vi "Generate_WayPoints_Hopping_CV_RunningAverage.vi"(11 "Input Cluster":T2={"Scan Rate (um/s)"=15.0, "X Start"=15.0, "X End"=15.0, "Y Start"=15.0, "Y End"=15.0, " Z Start"=15.0, "HoppingDistance"=1.0, "V"=15.0, "Z End"=15.0, "Approach Rate Hopping (um/s)"=15.0, "Retrack Rate (um/s)"=15.0, "V 2"=15.0, "Approach Rate (um/s)"=15.0, "V 3"=15.0, "CV Rate / V/s"=15.0, "V 4"=15.0, "V 1"=15.0, "HoldTime1/s"=15.0, "Hold time 2 / s"=15.0, "Hold time 3/ s"=15.0}) -> (0 "output cluster":T1)   [LabVIEW 2023]
uses:
  TypeDefs/WayPointCluster.ctl
  User_Vi/Settings.vi
panel:
  in  "WayPointCluster":T1
  out "Y  P":dbl
  out "X  P":dbl
  out "HoppingDistanceX":dbl
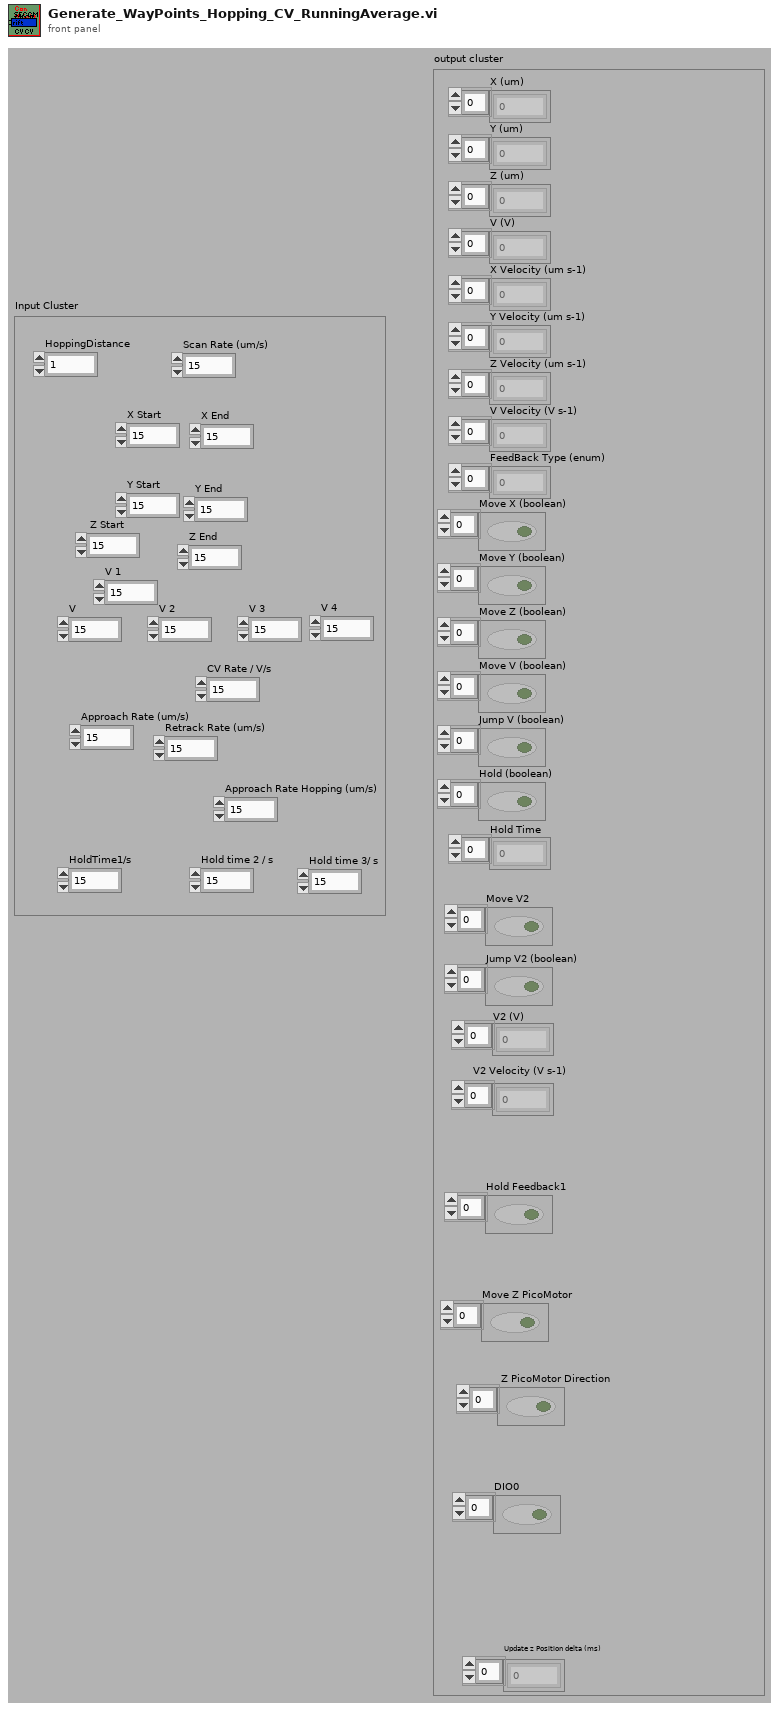
[diagram p1: front panel]
types:
  T1 = typedef "WayPointCluster.ctl" = cluster{"X (um)":dbl[], "Y (um)":dbl[], "Z (um)":dbl[], "V (V)":dbl[], "X Velocity (um s-1)":dbl[], "Y Velocity (um s-1)":dbl[], "Z Velocity (um s-1)":dbl[], "V Velocity (V s-1)":dbl[], "FeedBack Type (enum)":u16[], "Move X (boolean)":bool[], "Move Y (boolean)":bool[], "Move Z (boolean)":bool[], "Move V (boolean)":bool[], "Jump V (boolean)":bool[], "Hold (boolean)":bool[], "Hold Time":u32[], "V2 (V)":dbl[], "Move V2":bool[], "V2 Velocity (V s-1)":dbl[], "Jump V2 (boolean)":bool[], "Update z Position delta (ms)":i16[], "Hold Feedback1":bool[], "Move Z PicoMotor":bool[], " Z PicoMotor Direction":bool[], "DIO0":bool[]}
  T2 = cluster{"Scan Rate (um/s)":dbl, "X Start":dbl, "X End":dbl, "Y Start":dbl, "Y End":dbl, " Z Start":dbl, "HoppingDistance":dbl, "V":dbl, "Z End":dbl, "Approach Rate Hopping (um/s)":dbl, "Retrack Rate (um/s)":dbl, "V 2":dbl, "Approach Rate (um/s)":dbl, "V 3":dbl, "CV Rate / V/s":dbl, "V 4":dbl, "V 1":dbl, "HoldTime1/s":dbl, "Hold time 2 / s":dbl, "Hold time 3/ s":dbl}
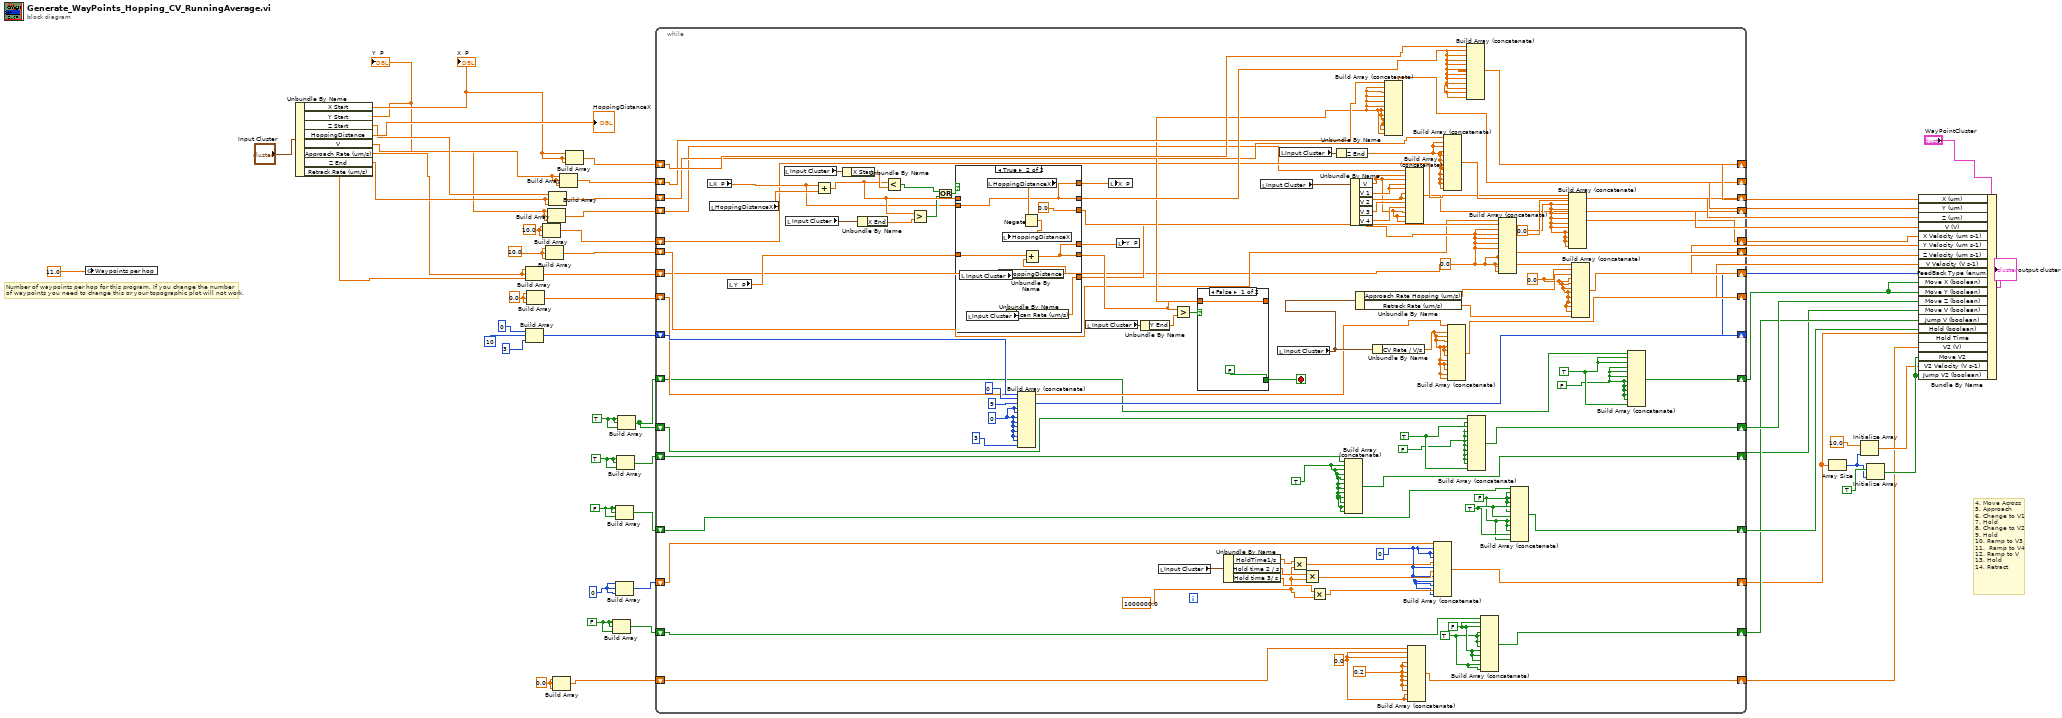
[diagram p0: block diagram]
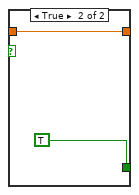
[diagram p2: hidden frame]
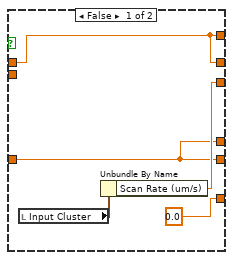
[diagram p3: hidden frame]
diagram:
  w4 = 0.0 ("element")
  w21 = FALSE
  w25 = FALSE
  w24 = u32 0 ("element")
  w23 = TRUE
  w19 = TRUE
  w15 = 10.0 ("element")
  w16 = 10.0 ("element")
  w18 = 0.0 ("element")
  # "Number of waypoints per hop for this program. If you change the number\nof waypoints you need to change this or your topographic plot will not work."
  # "4. Move Across\n5. Approach\n6. Change to V1\n7. Hold\n8. Change to V2\n9. Hold\n10. Ramp to V3\n11.  Ramp to V4\n12. Ramp to V\n13. Hold\n14. Retract"
  n1 = global write "Settings.vi" "Waypoints per hop"(11.0) -> ()
  n2 = Unbundle By Name("Input Cluster") -> ("X Start"=w39:dbl, "Y Start"=w38:dbl, "Z Start"=w40:dbl, "HoppingDistance"=→"HoppingDistanceX":dbl, "V"=w36:dbl, "Approach Rate (um/s)"=w17:dbl, "Z End"=w37:dbl, "Retrack Rate (um/s)"=w35:dbl)
  "X  P" <- w39
  "Y  P" <- w38
  n3 = Build Array(w17, w17, w35) -> (w47:dbl[])
  n4 = Build Array(u16 0 ("element"), u16 10 ("element"), u16 3 ("element")) -> (w43:u16[])
  n5 = Build Array(w18, w18, w18) -> (w45:dbl[])
  n6 = Build Array(w15, w15, w15) -> (w50:dbl[])
  n7 = Build Array(w16, w16, w16) -> (w49:dbl[])
  n8 = Build Array(w36, w36, w36) -> (w52:dbl[])
  n9 = Build Array(w40, w37, w37) -> (w54:dbl[])
  n10 = Build Array(w4, w4, w4) -> (w3:dbl[])
  n11 = Build Array(w38, w38, w38) -> (w56:dbl[])
  n12 = Build Array(w39, w39, w39) -> (w58:dbl[])
  n13 = Build Array(w25, w25, w25) -> (w29:bool[])
  n14 = Build Array(w21, w21, w21) -> (w20:bool[])
  n15 = Build Array(w24, w24, w24) -> (w32:u32[])
  n16 = Build Array(w23, w23, w23) -> (w27:bool[])
  n17 = Build Array(w19, w19, w19) -> (w11:bool[])
  n18 = while {
    shift-right: [w125] -> w57
    shift-left: w58 -> [w126]
    shift-right: [w122] -> w55
    shift-left: w56 -> [w123]
    shift-right: [w119] -> w53
    shift-left: w54 -> [w120]
    shift-right: [w109] -> w51
    shift-left: w52 -> [w110]
    shift-right: [w103] -> w33
    shift-left: w50 -> [w117]
    shift-right: [w112] -> w48
    shift-left: w49 -> [w113]
    shift-right: [w101] -> w46
    shift-left: w47 -> [w102]
    shift-right: [w96] -> w44
    shift-left: w45 -> [w97]
    shift-right: [w149] -> w42
    shift-left: w43 -> [w150]
    shift-right: [w93] -> w31
    shift-left: w11 -> [w94]
    shift-right: [w87] -> w30
    shift-left: w20 -> [w88]
    shift-right: [w83] -> w10
    shift-left: w32 -> [w84]
    shift-right: [w73] -> w28
    shift-left: w29 -> [w74]
    shift-right: [w90] -> w22
    shift-left: w27 -> [w91]
    shift-right: [w66] -> w12
    shift-left: w11 -> [w65]
    shift-right: [w63] -> w2
    shift-left: w3 -> [w64]
    stop <- w137 stop-if-true
    w62 = 0.2 ("element")
    w61 = 0.0 ("element")
    w68 = FALSE
    w69 = TRUE
    w70 = 1000000.0 ("y")
    w71 = TRUE
    w115 = 0.0 ("element")
    w89 = TRUE
    w72 = FALSE
    w75 = u32 0 ("element")
    w86 = TRUE
    w85 = FALSE
    w67 = FALSE
    w92 = TRUE
    w128 = u16 0 ("element")
    w111 = 0.0 ("element")
    w99 = 0.0 ("element")
    n19 = local read "X  P"() -> (w136:dbl)
    n20 = local read "HoppingDistanceX"() -> (w151:dbl)
    n21 = local read "Y  P"() -> (w135:dbl)
    n22 = local read "Input Cluster"() -> (w153:T2)
    n23 = local read "Input Cluster"() -> (w152:T2)
    n24 = Add(x=w136, y=w151) -> (x+y=w143:dbl)
    n25 = Unbundle By Name(w153) -> ("X Start"=w146:dbl)
    n26 = Unbundle By Name(w152) -> ("X End"=w144:dbl)
    n27 = Less?(x=w143, y=w146) -> (x < y?=w145:bool)
    n28 = Greater?(x=w143, y=w144) -> (0:w142:bool)
    n29 = Or(x=w145, y=w142) -> (x .or. y?=w141:bool)
    n30 = case shown="True" w141 {
      tunnel: w143 -> [w158 _]
      tunnel: [w158 w164] -> w124
      tunnel: w136 -> [_ w164]
      tunnel: w135 -> [w159 w165]
      tunnel: [w159 w163] -> w134
      tunnel: [w161 0.0] -> w116
      tunnel: [0.0 w166] -> w114
      tunnel: [w159 w163] -> w133
      tunnel: [w158 w164] -> w132
      frame False {
        n31 = local read "Input Cluster"() -> (w162:T2)
        n32 = Unbundle By Name(w162) -> ("Scan Rate (um/s)"=w161:dbl)
      }
      frame True {
        n33 = local read "Input Cluster"() -> (w170:T2)
        n34 = local read "Input Cluster"() -> (w168:T2)
        n35 = local read "HoppingDistanceX"() -> (w172:dbl)
        n36 = Unbundle By Name(w170) -> ("HoppingDistance"=w169:dbl)
        n37 = Unbundle By Name(w168) -> ("Scan Rate (um/s)"=w166:dbl)
        n38 = Negate(x=w172) -> (-x=w171:dbl)
        n39 = local write "HoppingDistanceX"(w171) -> ()
        n40 = Add(x=w165, y=w169) -> (x+y=w163:dbl)
      }
    }
    n41 = Build Array (concatenate)(w150, u16 0 ("element"), u16 9 ("element"), w128, w128, w128, w128, w128, w128, w128, w128, u16 3 ("element")) -> (w149:u16[])
    n42 = local read "Input Cluster"() -> (w140:T2)
    n43 = local write "X  P"(w132) -> ()
    n44 = local write "Y  P"(w133) -> ()
    n45 = Unbundle By Name(w140) -> ("Y End"=w139:dbl)
    n46 = local read "Input Cluster"() -> (w82:T2)
    n47 = Greater?(x=w134, y=w139) -> (0:w138:bool)
    n48 = case shown="False" w138 {
      tunnel: w134 -> [w155 w157]
      tunnel: [w155 w157] -> w121
      tunnel: [FALSE TRUE] -> w137
      frame False {
      }
      frame True {
      }
    }
    n49 = Unbundle By Name(w82) -> ("HoldTime1/s"=w81:dbl, "Hold time 2 / s"=w80:dbl, "Hold time 3/ s"=w79:dbl)
    n50 = local read "Input Cluster"() -> (w147:T2)
    n51 = local read "Input Cluster"() -> (w129:T2)
    n52 = local read "Input Cluster"() -> (w148:T2)
    n53 = Multiply(x=w81, y=w70) -> (x*y=w78:dbl)
    n54 = Multiply(x=w80, y=w70) -> (x*y=w77:dbl)
    n55 = Multiply(x=w79, y=w70) -> (x*y=w76:dbl)
    n56 = Unbundle By Name(w148) -> ("Z End"=w118:dbl)
    n57 = Build Array (concatenate)(w91, w89, w89, w89, w89, w89, w89, w89, w89, w89, w89, w89) -> (w90:bool[])
    n58 = Unbundle By Name(w147) -> ("V"=w104:dbl, "V 1"=w108:dbl, "V 2"=w107:dbl, "V 3"=w106:dbl, "V 4"=w105:dbl)
    n59 = Unbundle By Name(w129) -> ("Approach Rate Hopping (um/s)"=w100:dbl, "Retrack Rate (um/s)"=w98:dbl)
    n60 = Unbundle By Name(w129) -> ("CV Rate / V/s"=w95:dbl)
    n61 = Build Array (concatenate)(w123, w121, w121, w121, w121, w121, w121, w121, w121, w121, w121, w121) -> (w122:dbl[])
    n62 = Build Array (concatenate)(w110, w104, w104, w108, w108, w107, w107, w106, w105, w104, w104, w104) -> (w109:dbl[])
    n63 = Build Array (concatenate)(w64, w61, w61, w62, w62, w62, w62, w62, w62, w62, w61, w61) -> (w63:dbl[])
    n64 = Build Array (concatenate)(w84, w75, w75, w75, w78, w75, w77, w75, w75, w75, w76, w75) -> (w83:dbl[])
    n65 = Build Array (concatenate)(w120, w118, w118, w118, w118, w118, w118, w118, w118, w118, w118, w118) -> (w119:dbl[])
    n66 = Build Array (concatenate)(w97, w95, w95, w95, w95, w95, w95, w95, w95, w95, w95, w95) -> (w96:dbl[])
    n67 = Build Array (concatenate)(w126, w124, w124, w124, w124, w124, w124, w124, w124, w124, w124, w124) -> (w125:dbl[])
    n68 = Build Array (concatenate)(w94, w67, w92, w67, w67, w67, w67, w67, w67, w67, w67, w92) -> (w93:bool[])
    n69 = Build Array (concatenate)(w74, w72, w72, w71, w71, w71, w71, w72, w72, w72, w71, w71) -> (w73:bool[])
    n70 = Build Array (concatenate)(w113, w114, w111, w111, w111, w111, w111, w111, w111, w111, w111, w111) -> (w112:dbl[])
    n71 = Build Array (concatenate)(w88, w85, w85, w85, w86, w85, w86, w85, w85, w85, w86, w85) -> (w87:bool[])
    n72 = Build Array (concatenate)(w117, w116, w115, w115, w115, w115, w115, w115, w115, w115, w115, w115) -> (w103:dbl[])
    n73 = Build Array (concatenate)(w102, w99, w100, w99, w99, w99, w99, w99, w99, w99, w99, w98) -> (w101:dbl[])
    n74 = Build Array (concatenate)(w65, w69, w69, w68, w68, w68, w68, w68, w68, w68, w68, w69) -> (w66:bool[])
  }
  n75 = Array Size(array=w10) -> (size(s)=w7:i32)
  n76 = Initialize Array(10.0 ("element"), w7) -> (w5:dbl[])
  n77 = Initialize Array(TRUE, w7) -> (w8:bool[])
  n78 = Bundle By Name(cluster="WayPointCluster", "X (um)"=w57, "Y (um)"=w55, "Z (um)"=w53, "V (V)"=w51, "X Velocity (um s-1)"=w33, "Y Velocity (um s-1)"=w48, "Z Velocity (um s-1)"=w46, "V Velocity (V s-1)"=w44, "FeedBack Type (enum)"=w42, "Move X (boolean)"=w12, "Move Y (boolean)"=w12, "Move Z (boolean)"=w31, "Move V (boolean)"=w22, "Jump V (boolean)"=w28, "Hold (boolean)"=w30, "Hold Time"=w10, "V2 (V)"=w2, "Move V2"=w8, "V2 Velocity (V s-1)"=w5, "Jump V2 (boolean)"=w8) -> (→"output cluster":T1)
